vi "Send OCP Settings.vi"(8 "error in":errorcluster, 10 "Channel List":T1, 11 "Electronic Load in":refnum<class "Electronic Load.lvclass">) -> (0 "error out":errorcluster, 3 "Electronic Load out":refnum<class "Electronic Load.lvclass">)   [LabVIEW 2019]
uses:
  Electronic Load.lvclass
  Custom Controls/Value to Send.ctl
  Custom Controls/Channel Select.ctl
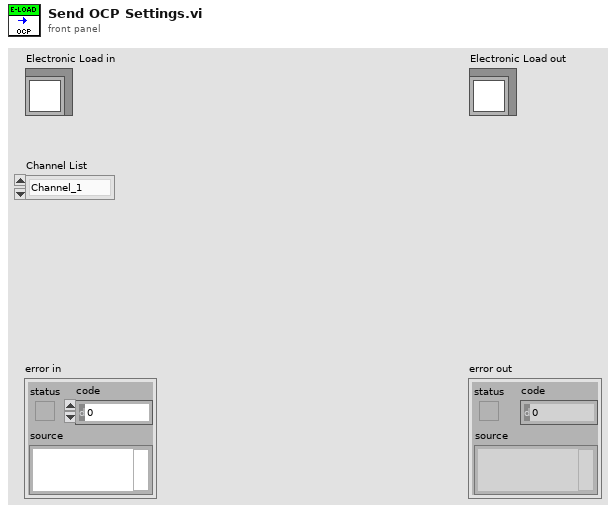
[diagram p1: front panel]
types:
  T1 = typedef "Electronic Load.lvlib/Electronic Load.lvclass/Channel Select.ctl" = enum16{"Channel_1", "Channel_2", "Channel_3", "Channel_4", "Channel_5", "Channel_6"}
  T2 = typedef "Electronic Load.lvlib/Electronic Load.lvclass/Value to Send.ctl" = enum16{"Trigger - Enable", "Trigger - Sample Interval", "Trigger - Data Points", "Trigger - Current(Initial)", "Trigger - Transient Current", "Trigger - Pulse Width", "Trigger - Delay", "OCP - Enable", "OCP - Level", "OCP - Delay", "Function - Mode", "Function - Value", "Function - Enabled"}
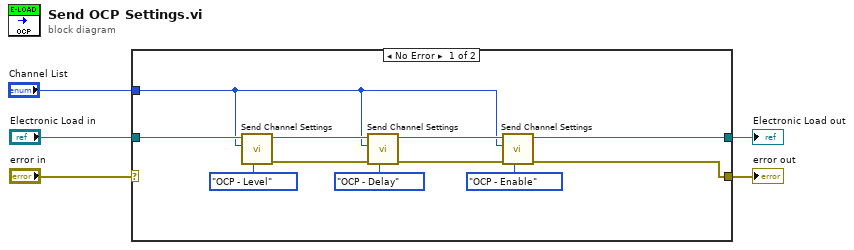
[diagram p0: block diagram]
diagram:
  n1 = case shown="No Error" "error in" {
    selector: "error in" -> [_ w18]
    tunnel: [w7 w18] -> w4
    tunnel: [w10 w17] -> w2
    tunnel: "Electronic Load in" -> [w16 w17]
    tunnel: "Channel List" -> [w6 _]
    frame No Error {
      n2 = call-dynamic "Send Channel Settings.vi"("Value to Send"=Value_to_Send."OCP - Level", "Channel List"=w6, "Electronic Load in"=w16) -> ("error out"=w9:errorcluster, "Electronic Load out"=w12:refnum<class "Electronic Load.lvclass">)  [unwired: 7 in]
      n3 = call-dynamic "Send Channel Settings.vi"("Value to Send"=Value_to_Send."OCP - Delay", "error in (no error)"=w9, "Channel List"=w6, "Electronic Load in"=w12) -> ("error out"=w8:errorcluster, "Electronic Load out"=w11:refnum<class "Electronic Load.lvclass">)  [unwired: 6 in]
      n4 = call-dynamic "Send Channel Settings.vi"("Value to Send"=Value_to_Send."OCP - Enable", "error in (no error)"=w8, "Channel List"=w6, "Electronic Load in"=w11) -> ("error out"=w7:errorcluster, "Electronic Load out"=w10:refnum<class "Electronic Load.lvclass">)  [unwired: 6 in]
    }
    frame Error {
    }
  }
  "error out" <- w4
  "Electronic Load out" <- w2
